vi "Read mode.vi"(8 "error in (no error)":errorcluster, 11 "WSMode.lvclass in":refnum<class "WSMode.lvclass">) -> (0 "error out":errorcluster, 2 "wsMode":T1, 3 "WSMode.lvclass out":refnum<class "WSMode.lvclass">)   [LabVIEW 2014, in "TCSDataDefinitions.lvlib" / "TCSWeatherServerCommand.lvlib" / "WSMode.lvclass"]
uses:
  WSMode.lvclass
  Enumerations/wsMode.ctl
  WSMode.lvclass/WSMode.ctl
  TCSWeatherServerCommand.lvlib
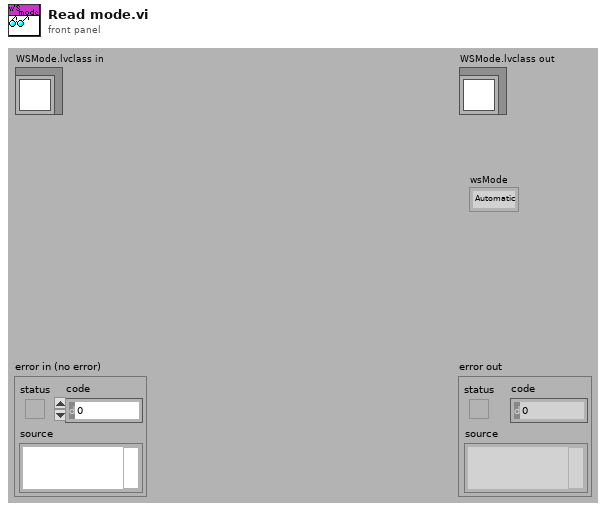
[diagram p1: front panel]
types:
  T1 = typedef "TCSDataDefinitions.lvlib/TCSWeatherServerCommand.lvlib/wsMode.ctl" = enum16{"Automatic", "Manual"}
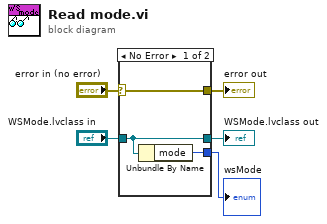
[diagram p0: block diagram]
diagram:
  n1 = case shown="No Error" "error in (no error)" {
    selector: "error in (no error)" -> [w8 w9]
    tunnel: [w8 w9] -> w4
    tunnel: [w7 w10] -> w2
    tunnel: "WSMode.lvclass in" -> [w7 w10]
    tunnel: [w6 _] -> w1
    frame No Error {
      n2 = Unbundle By Name(w7) -> ("mode"=w6:T1)
    }
    frame Error {
    }
  }
  "error out" <- w4
  "WSMode.lvclass out" <- w2
  "wsMode" <- w1
